vi "DVS_LabVIEWController_one_panel.vi"() -> ()   [LabVIEW 2013]
doc: "This example demonstrates temperature control and monitoring.\n\nNote:\nBefore start this VI is it necessary:\n\n- preconfigure some specific parameters that are not supported by this driver (e.g. PV-I/O Type, Linearization type, Alarm Input Values... ) by Quick Codes, or by Eurotherm iTools or by instrument front panel controls\n- enter correct VISA Resource Descriptor, Device Address and Baud Rate into front-panel controls"
uses:
  <vilib>/Utility/file.llb/Write To Spreadsheet File (string).vi
  <vilib>/Instr/_visa.llb/VISA Configure Serial Port (Instr).vi
  <instrlib>/Keithley 24XX/Public/Data/Read (Single Point).vi
  <instrlib>/Keithley 24XX/Keithley 24XX.lvlib
panel:
  out "Data\nfile\npath":path
  in  "4-wire?":bool
  in  "stop":bool
  in  "Add comments to the   here and click anywhere outside\nthe comment box to save. The time at which the comment is\nsaved is recorded in the data file.":string
  in  "O2 PUMP":bool
  in  "QCM":bool
  in  "Keithley 2420":bool
  in  "J-KEM":bool
  in  "RapidOX":bool
  out "Starting Time":string
  out "Time Elapsed (min)":dbl caption="Elapsed Time (s)"
  in  "Delay Between\nData Points (s)":dbl format="%#_13g"
  in  "Stop after":dbl
  in  "Automatically stop\nmeasurement?":bool
  out "min remaining":dbl
  out "Program Errors":errorcluster
  out "Freq (Hz)":dbl format="%.3e"
  out "R (Ohm)":dbl format="%.3e"
  out "Waveform Chart 7":T1(graph)
  out "Current Temp (C)":dbl
  in  "Setpoint (C)":dbl=25.0
  out "Current Setpoint (C)":dbl
  out "Waveform Chart 5":cluster{dbl, dbl}(graph)
  out "Waveform Chart":cluster{dbl}(graph)
  out "Torr":dbl
  out "%":dbl
  out "atm":dbl
  in  "Com Port":i32(ring) items=["Com 1", "Com 2", "Com 3", "Com 4", "Com 5", "Com 6", "COM 7", "COM 8", "COM 9", "COM 10", "COM 11", "COM 12", "com 13", "COM 14"]
  in  "Baud Rate 2":i32(ring)=2 items=["2400", "4800", "9600", "19200", "38400", "57600", "115200"]
  in  "Com Port 2":i32(ring) items=["Com 1", "Com 2", "Com 3", "Com 4", "Com 5", "Com 6", "COM 7", "COM 8", "COM 9", "COM 10", "COM 11", "COM 12", "com 13", "COM 14"]
  out "Waveform Chart 6":cluster{dbl}(graph)
  out "O2 Concentration (PPM)":dbl
  out "Resistance (Ohm)":sgl
  out "Waveform Chart 4":cluster{"Resistance":sgl}(graph)
  # "Keithley 2420\nRead Resistance"
  # "Setup"
  # "SRS QCM\nController"
  # "Instruments Connected:"
  # "Timing"
  # "Configuring Instrument\n \nPlease Wait......\n\nChart will update in 20 sec"
  # "min"
  # "COMMENT BOX"
  # "J-Kem Temp Control"
  # "Rapidox O2\nSensor"
  # "O2 Partial Pressure"
  # "SetNag\nO2 Pump"
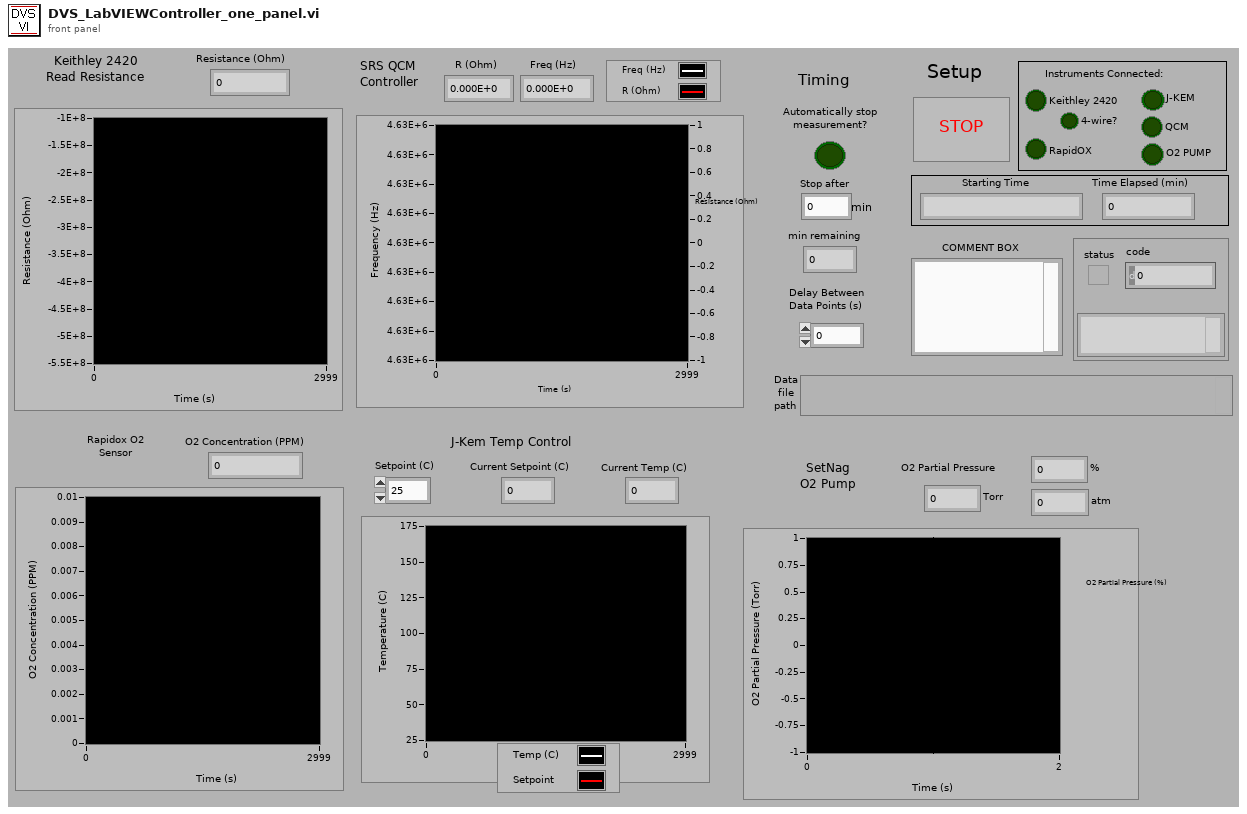
[diagram p1: front panel]
types:
  T1 = cluster{"Frequency out":dbl, "Resistance out":dbl}
  T2 = enum16{"open", "open or create", "create or replace", "create", "open (read only)"}
  T3 = enum16{"no parity", "odd parity", "even parity", "mark parity", "space parity"}
  T4 = cluster{bool, "VISA resource name":refnum<visa-resource-name>, "error out":errorcluster}
  T5 = cluster{bool, "VISA resource name out":refnum<visa-resource-name>, "error out":errorcluster}
  T6 = cluster{"Frequency out":dbl, "Resistance out":dbl}[]
  T7 = cluster{bool, "VISA out":refnum<visa-resource-name>, "error out":errorcluster}
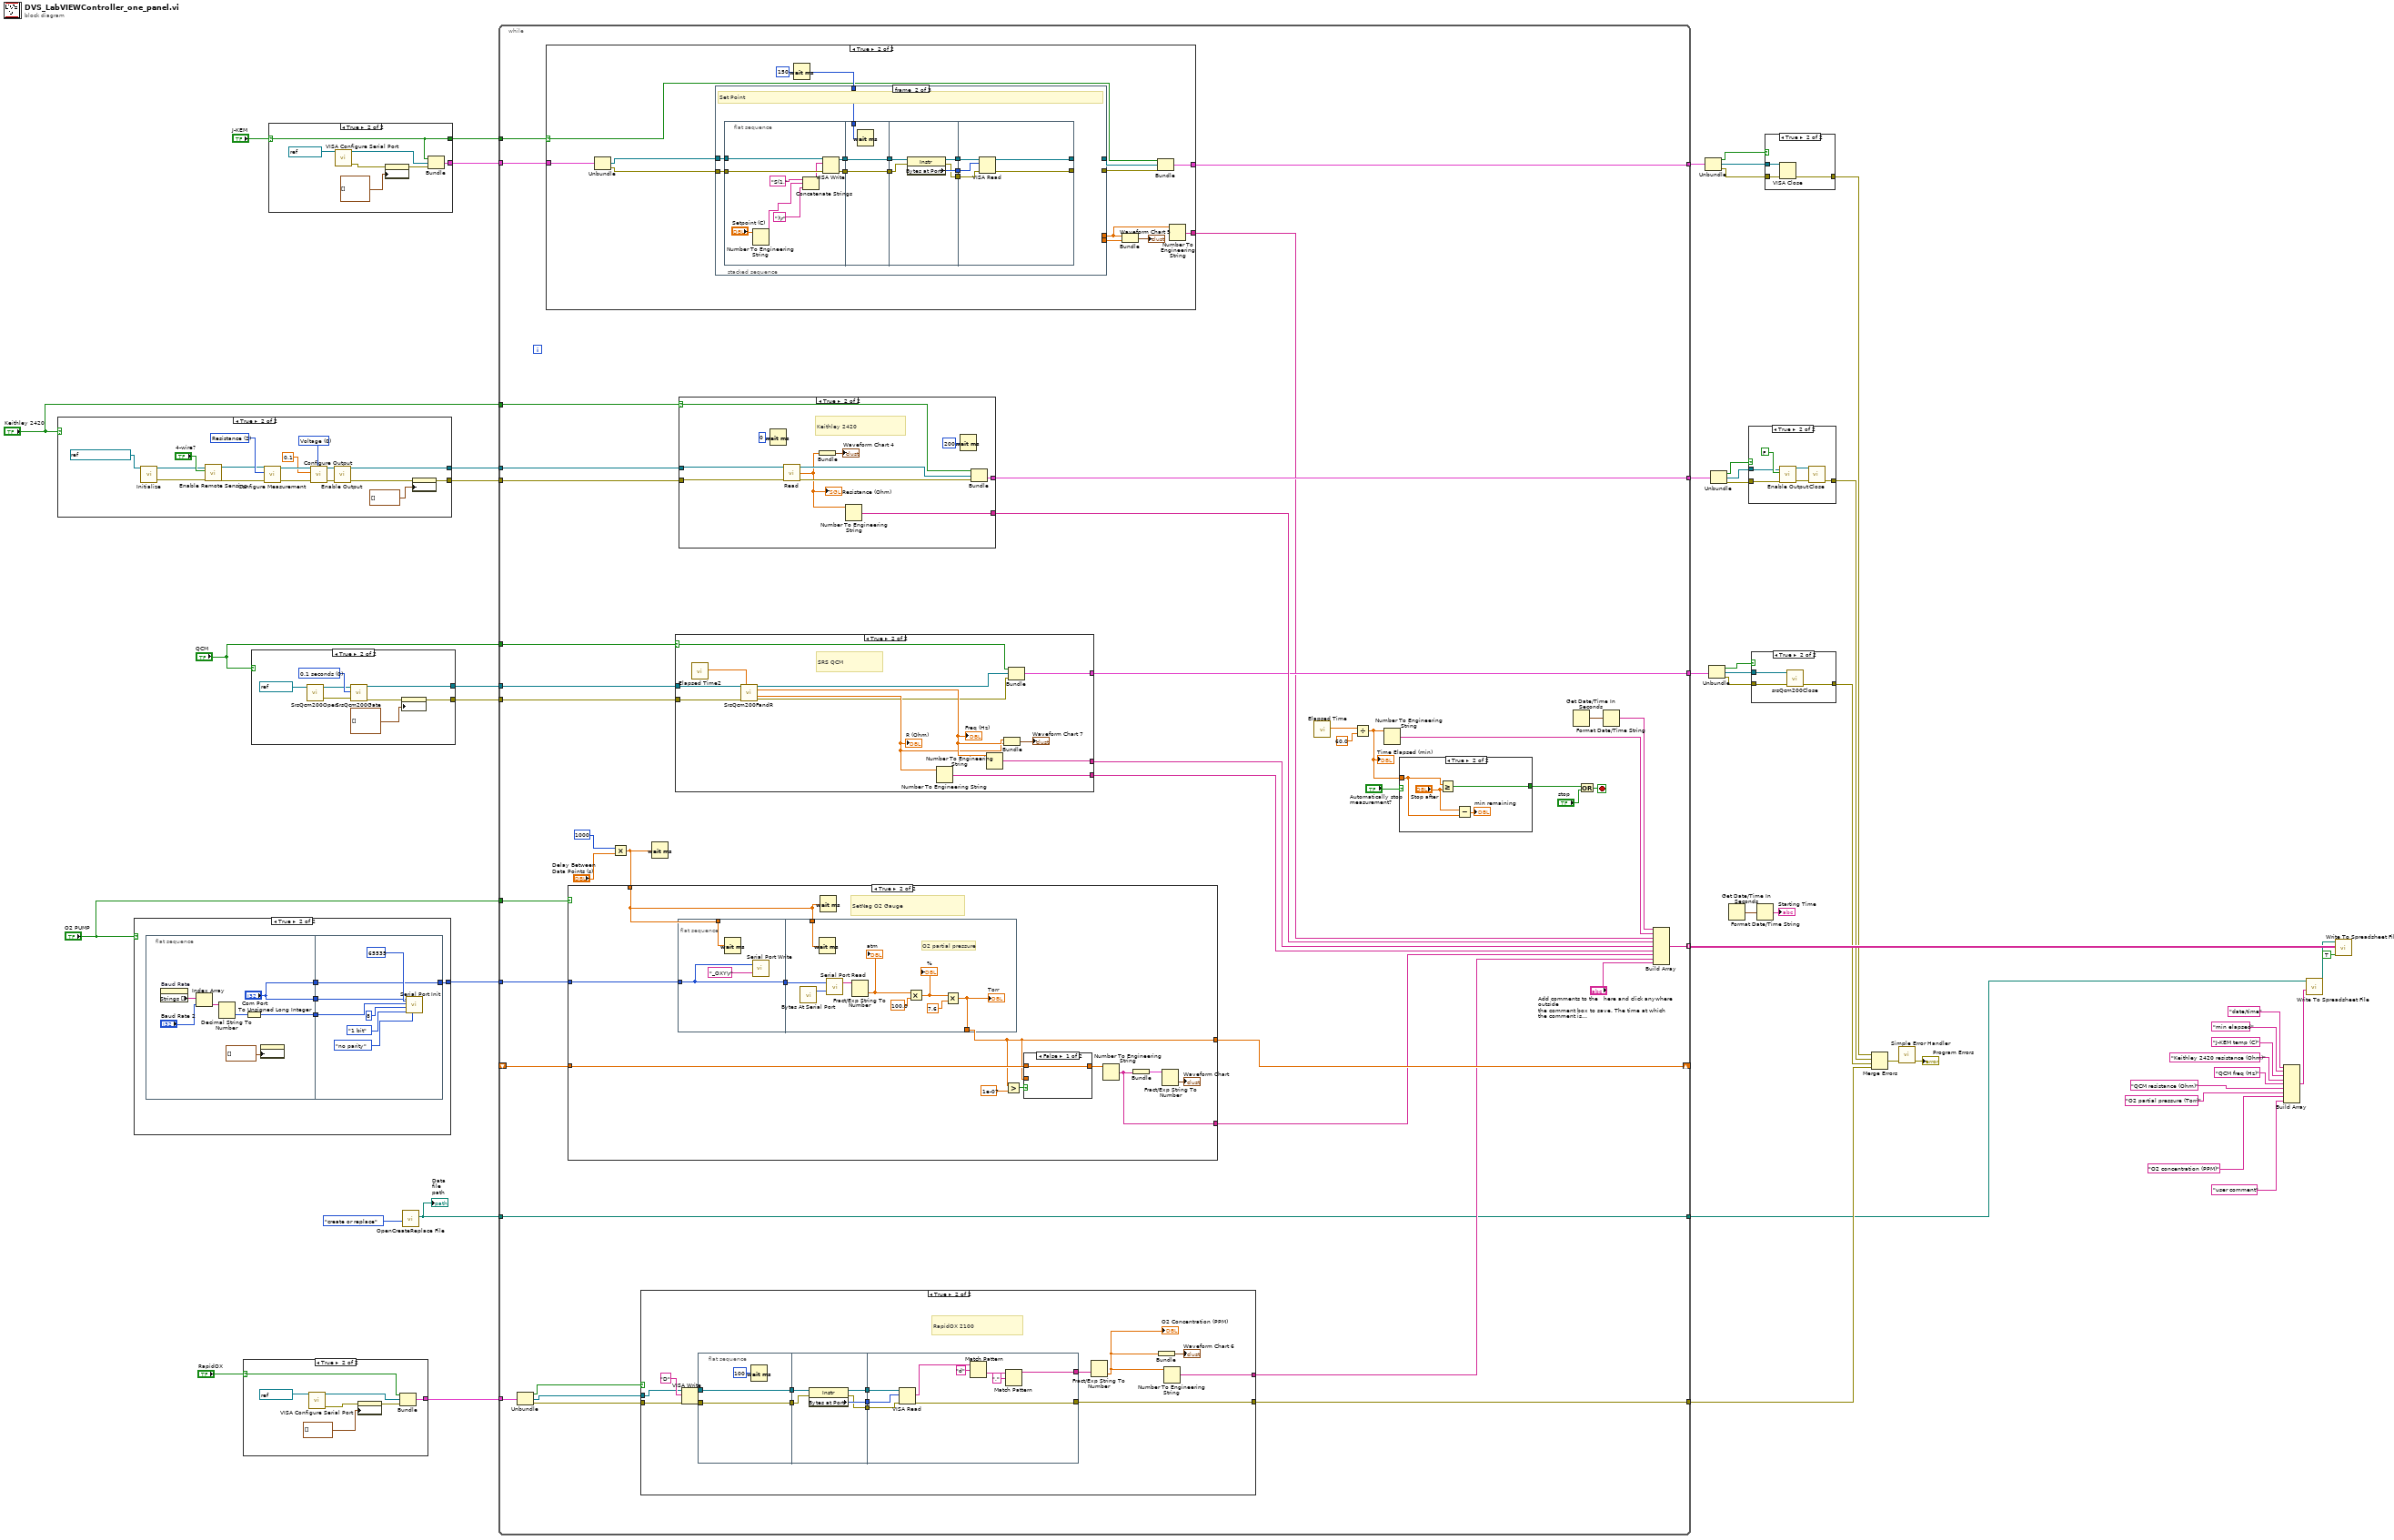
[diagram p0: block diagram]
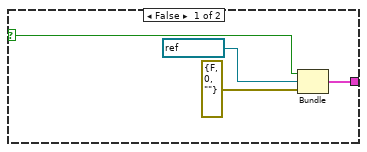
[diagram p2: hidden frame]
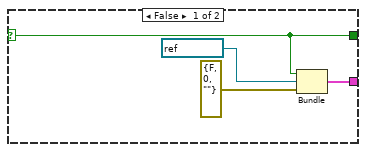
[diagram p4: hidden frame]
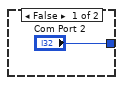
[diagram p5: hidden frame]
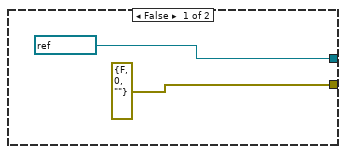
[diagram p7: hidden frame]
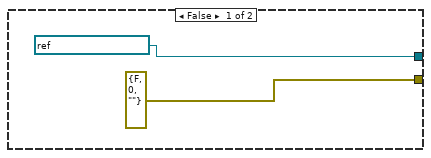
[diagram p9: hidden frame]
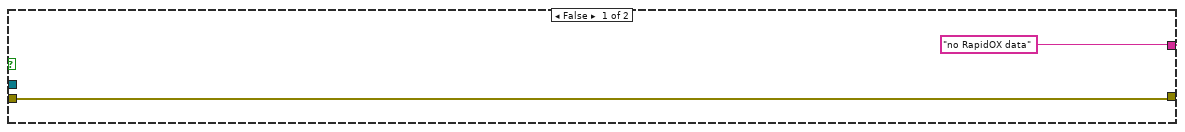
[diagram p10: hidden frame]
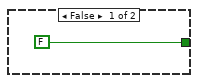
[diagram p11: hidden frame]
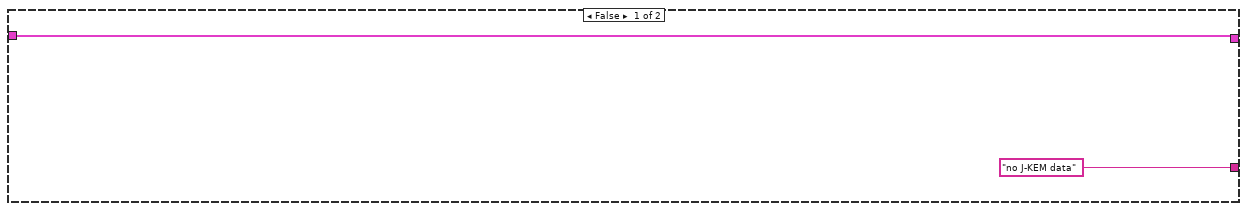
[diagram p12: hidden frame]
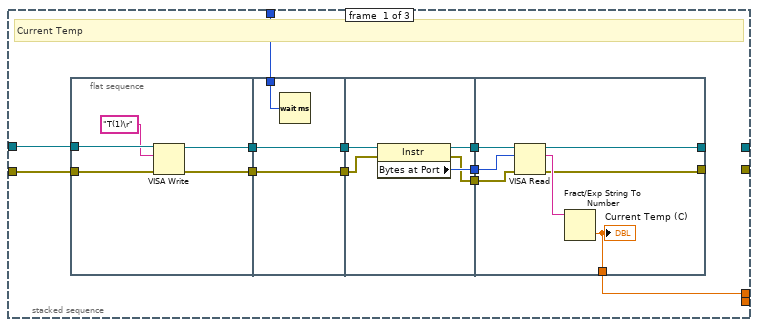
[diagram p13: hidden frame]
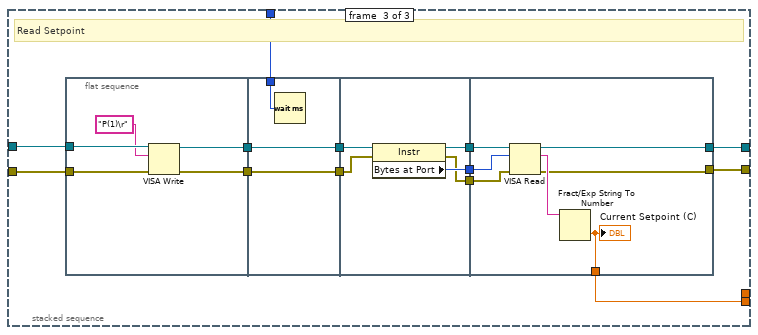
[diagram p14: hidden frame]
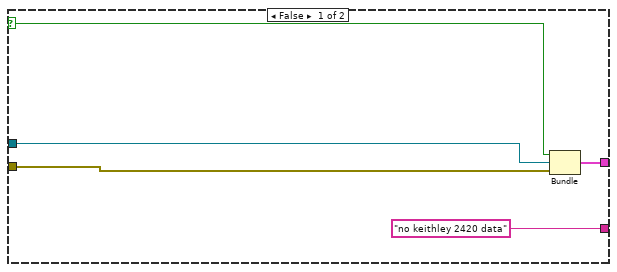
[diagram p15: hidden frame]
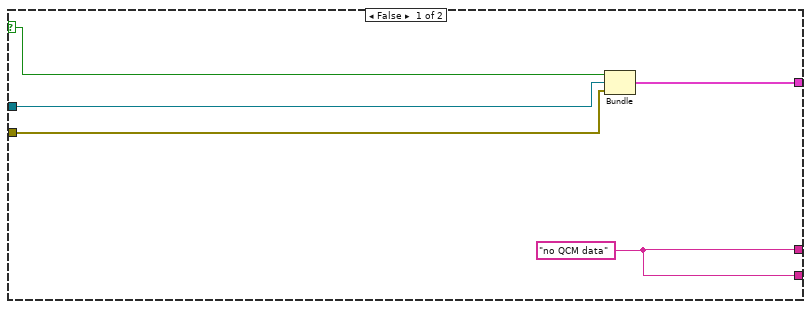
[diagram p16: hidden frame]
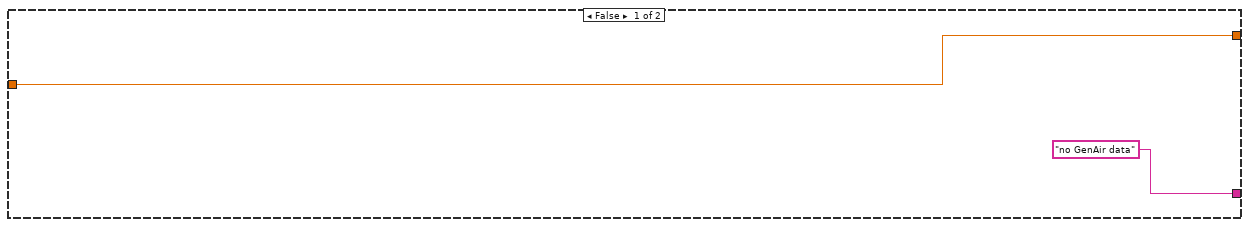
[diagram p17: hidden frame]
diagram:
  n1 = case shown="True" "Keithley 2420" {
    tunnel: [refnum<visa-resource-name> "GPIB1::24::INSTR" ("VISA resource name") w56] -> w43
    tunnel: [errorcluster {"status"=FALSE, "code"=0, "source"=""} ("error out") w59] -> w42
    frame False {
    }
    frame True {
      w62 = u16 0 items=["Voltage", "Current"] ("Source Mode  (0: Voltage)")
      w67 = u16 2 items=["Volts", "Current", "Resistance"] ("Function (0: Volts)")
      n2 = call <instrlib>:"Initialize.vi"("VISA resource name"=refnum<visa-resource-name> "GPIB1::24::INSTR") -> ("error out"=w52:errorcluster, "VISA resource name out"=w55:refnum<visa-resource-name>)  [unwired: 9 in]
      n3 = call <instrlib>:"Enable Remote Sensing.vi"("error in (no error)"=w52, "Enable Remote Sensing (T: Enable)"="4-wire?", "VISA resource name"=w55) -> ("error out"=w53:errorcluster, "VISA resource name out"=w54:refnum<visa-resource-name>)  [unwired: 7 in]
      n4 = call <instrlib>:"Configure Measurement.vi"("error in (no error)"=w53, "Function (0: Volts)"=w67, "VISA resource name"=w54) -> ("error out"=w66:errorcluster, "VISA resource name out"=w65:refnum<visa-resource-name>)  [unwired: 7 in]
      n5 = call <instrlib>:"Configure Output.vi"("Source Mode  (0: Voltage)"=w62, "error in (no error)"=w66, "Output Level (0)"=0.1 ("Output Level (V)"), "VISA resource name"=w65) -> ("error out"=w64:errorcluster, "VISA resource name out"=w63:refnum<visa-resource-name>)  [unwired: 6 in]
      n6 = call <instrlib>:"Enable Output.vi"("error in (no error)"=w64, "VISA resource name"=w63) -> ("error out"=w57:errorcluster, "VISA resource name out"=w56:refnum<visa-resource-name>)  [unwired: 8 in]
      n7 = property on="Waveform Chart 4" class="WFChart (strict)"(error in=w57, "History Data"=cluster{"Resistance":sgl}[] []) -> (error out=w59:errorcluster)  [unwired: 1 in, 1 out]
    }
  }
  n8 = case shown="True" "O2 PUMP" {
    tunnel: ["Com Port 2" w70] -> w37
    frame False {
    }
    frame True {
      n9 = flat-sequence {
        tunnel: ["Com Port"] -> w73
        tunnel: [w76] -> w72
        tunnel: ["Com Port"] -> w71
        tunnel: w73 -> [w82]
        tunnel: w72 -> [w81]
        tunnel: w71 -> [w83]
        tunnel: [w83] -> w70
        frame #0 {
          n10 = property on="Baud Rate" class="Ring (strict)"() -> ("Strings []"=w78:string[])  [unwired: 2 in, 2 out]
          n11 = Index Array(array=w78, index="Baud Rate 2") -> (element=w79:string)
          n12 = Decimal String To Number(string=w79) -> (number=w77:i32)  [unwired: 2 in, 1 out]
          n13 = To Unsigned Long Integer(number=w77) -> (unsigned 32bit integer=w76:u32)
          n14 = property on="Waveform Chart" class="WFChart (strict)"("History Data"=cluster{dbl}[] []) -> ()  [unwired: 2 in, 2 out]
        }
        frame #1 {
          n15 = call <vilib>:"Serial Port Init.vi"("parity"=T3."no parity", "buffer size"=u16 65535, "stop bits"=enum16{"1 bit", "1.5 bits", "2 bits"}."1 bit", "data bits"=u16 8, "baud rate"=w81, "port number"=w82) -> ()  [unwired: 1 in, 1 out]
        }
      }
    }
  }
  n16 = case shown="True" "RapidOX" {
    selector: "RapidOX" -> [w88 w95]
    tunnel: [w89 w96] -> w5
    frame False {
      n17 = Bundle(w88, "VISA resource name"=refnum<visa-resource-name> "COM7", "error out"=errorcluster {"status"=FALSE, "code"=0, "source"=""}) -> (w89:T4)  [unwired: 1 in]
    }
    frame True {
      n18 = call-poly "VISA Configure Serial Port"("VISA resource name"=refnum<visa-resource-name> "COM7") -> ("VISA resource name out"=w97:refnum<visa-resource-name>, "error out"=w93:errorcluster)  [unwired: 13 in]
      n19 = property on="Waveform Chart 6" class="WFChart (strict)"(error in=w93, "History Data"=cluster{dbl}[] []) -> (error out=w92:errorcluster)  [unwired: 1 in, 1 out]
      n20 = Bundle(w95, "VISA resource name out"=w97, "error out"=w92) -> (w96:T5)  [unwired: 1 in]
    }
  }
  n21 = case shown="True" "QCM" {
    tunnel: [refnum<visa-resource-name> "COM6" ("VISA in") w104] -> w41
    tunnel: [errorcluster {"status"=FALSE, "code"=0, "source"=""} ("error out") w102] -> w40
    frame False {
    }
    frame True {
      w108 = u16 0 items=["0.1 seconds", "1.0 seconds", "10.0 seconds"] ("Gate in")
      n22 = call <instrlib>:"SrsQcm200Open.vi"("VISA in"=refnum<visa-resource-name> "COM6") -> ("error out"=w105:errorcluster, "VISA out"=w106:refnum<visa-resource-name>)  [unwired: 4 in]
      n23 = call <instrlib>:"SrsQcm200Gate.vi"("VISA in"=w106, "Gate in"=w108, "error in (no error)"=w105) -> ("VISA out"=w104:refnum<visa-resource-name>, "error out"=w101:errorcluster)  [unwired: 14 in, 1 out]
      n24 = property on="Waveform Chart 7" class="WFChart (strict)"(error in=w101, "History Data"=T6 []) -> (error out=w102:errorcluster)  [unwired: 1 in, 1 out]
    }
  }
  n25 = case shown="True" "J-KEM" {
    selector: "J-KEM" -> [w109 w116]
    tunnel: [w110 w117] -> w26
    tunnel: [w109 w116] -> w19
    frame False {
      n26 = Bundle(w109, "VISA resource name"=refnum<visa-resource-name> "COM3", "error out"=errorcluster {"status"=FALSE, "code"=0, "source"=""}) -> (w110:T4)  [unwired: 1 in]
    }
    frame True {
      n27 = call-poly "VISA Configure Serial Port"("VISA resource name"=refnum<visa-resource-name> "COM3") -> ("VISA resource name out"=w118:refnum<visa-resource-name>, "error out"=w114:errorcluster)  [unwired: 13 in]
      n28 = property on="Waveform Chart 5" class="WFChart (strict)"(error in=w114, "History Data"=cluster{dbl, dbl}[] []) -> (error out=w113:errorcluster)  [unwired: 1 in, 1 out]
      n29 = Bundle(w116, "VISA resource name out"=w118, "error out"=w113) -> (w117:T5)  [unwired: 1 in]
    }
  }
  n30 = call <instrlib>:"OpenCreateReplace File.vi"("function (open:0)"=T2."create or replace") -> ("new file path"=w1:path)  [unwired: 7 in, 3 out]
  "Data\nfile\npath" <- w1
  n31 = while {
    shift-right: [w159] -> _
    shift-left: _ -> [w158]
    tunnel: [w156] -> w45 mode=indexing
    tunnel: "Keithley 2420" -> [w122]
    tunnel: w43 -> [w154]
    tunnel: w42 -> [w153]
    tunnel: w41 -> [w152]
    tunnel: w40 -> [w151]
    tunnel: "QCM" -> [w149]
    tunnel: "O2 PUMP" -> [w142]
    tunnel: w37 -> [w148]
    tunnel: [w144] -> w34
    tunnel: [w143] -> w30
    tunnel: w26 -> [w141]
    tunnel: [w140] -> w24
    tunnel: w19 -> [w138]
    tunnel: w5 -> [w131]
    tunnel: [w126] -> w3
    tunnel: [w120] -> w2
    tunnel: w1 -> [w120]
    stop <- w136 stop-if-true
    n32 = Unbundle(w131) -> (w130:bool, "VISA resource name out"=w129:refnum<visa-resource-name>, "error out"=w128:errorcluster)
    n33 = case shown="True" w138 {
      selector: w138 -> [_ w204]
      tunnel: w141 -> [w202 w209]
      tunnel: [w202 w207] -> w140
      tunnel: ["no J-KEM data" w205] -> w139
      frame False {
      }
      frame True {
        w214 = u32 150 ("milliseconds to wait")
        n34 = Unbundle(w209) -> ("VISA resource name out"=w208:refnum<visa-resource-name>, "error out"=w203:errorcluster)  [unwired: 1 out]
        n35 = stacked-sequence {
          tunnel: w208 -> [w218 w248 w282]
          tunnel: w203 -> [w217 w247 w281]
          tunnel: w214 -> [w216 w246 w283]
          tunnel: [_ _ w280] -> w210
          tunnel: [_ _ w279] -> w211
          tunnel: [w215 _ _] -> w206
          tunnel: [_ _ w278] -> w213
          frame #0 {
            # "Current Temp"
            n36 = flat-sequence {
              tunnel: w218 -> [w230]
              tunnel: w217 -> [w229]
              tunnel: [w227] -> w225
              tunnel: [w226] -> w224
              tunnel: w216 -> [w233]
              tunnel: [w232] -> w223
              tunnel: w225 -> [w232]
              tunnel: w224 -> [w231]
              tunnel: [w231] -> w222
              tunnel: w223 -> [w238]
              tunnel: w222 -> [w237]
              tunnel: [w236] -> w221
              tunnel: [w235] -> w220
              tunnel: [w234] -> w219
              tunnel: w221 -> [w245]
              tunnel: w220 -> [w244]
              tunnel: w219 -> [w243]
              tunnel: [w240] -> _
              tunnel: [w241] -> _
              tunnel: [w239] -> w215
              frame #0 {
                n37 = VISA Write(VISA resource name=w230, write buffer="T(1)\r", error in (no error)=w229) -> (VISA resource name out=w227:refnum<visa-resource-name>, error out=w226:errorcluster)  [unwired: 1 out]
              }
              frame #1 {
                n38 = Wait (ms)(milliseconds to wait=w233) -> ()  [unwired: 1 out]
              }
              frame #2 {
                n39 = property class="Instr"(reference=w238, error in=w237) -> (reference out=w236:refnum<visa-resource-name>, error out=w234:errorcluster, "Bytes at Port"=w235:u32)
              }
              frame #3 {
                n40 = VISA Read(VISA resource name=w245, byte count=w244, error in (no error)=w243) -> (VISA resource name out=w241:refnum<visa-resource-name>, read buffer=w242:string, error out=w240:errorcluster)  [unwired: 1 out]
                n41 = Fract/Exp String To Number(string=w242) -> (number=w239:dbl)  [unwired: 3 in, 1 out]
                "Current Temp (C)" <- w239
              }
            }
          }
          frame #1 {
            # "Set Point"
            n42 = flat-sequence {
              tunnel: w248 -> [w264]
              tunnel: w247 -> [w263]
              tunnel: [w262] -> w255
              tunnel: [w261] -> w254
              tunnel: w246 -> [w267]
              tunnel: [w266] -> w253
              tunnel: w255 -> [w266]
              tunnel: w254 -> [w265]
              tunnel: [w265] -> w252
              tunnel: w253 -> [w272]
              tunnel: w252 -> [w271]
              tunnel: [w270] -> w251
              tunnel: [w269] -> w250
              tunnel: [w268] -> w249
              tunnel: w251 -> [w277]
              tunnel: w250 -> [w276]
              tunnel: w249 -> [w275]
              tunnel: [w273] -> _
              tunnel: [w274] -> _
              frame #0 {
                n43 = Number To Engineering String(4:"Setpoint (C)") -> (0:w257:string)  [unwired: 3 in]
                n44 = Concatenate Strings("S(1," ("write buffer"), w257, ")\r" ("write buffer")) -> (w260:string)
                n45 = VISA Write(VISA resource name=w264, write buffer=w260, error in (no error)=w263) -> (VISA resource name out=w262:refnum<visa-resource-name>, error out=w261:errorcluster)  [unwired: 1 out]
              }
              frame #1 {
                n46 = Wait (ms)(milliseconds to wait=w267) -> ()  [unwired: 1 out]
              }
              frame #2 {
                n47 = property class="Instr"(reference=w272, error in=w271) -> (reference out=w270:refnum<visa-resource-name>, error out=w268:errorcluster, "Bytes at Port"=w269:u32)
              }
              frame #3 {
                n48 = VISA Read(VISA resource name=w277, byte count=w276, error in (no error)=w275) -> (VISA resource name out=w274:refnum<visa-resource-name>, error out=w273:errorcluster)  [unwired: 2 out]
              }
            }
          }
          frame #2 {
            # "Read Setpoint"
            n49 = flat-sequence {
              tunnel: w282 -> [w295]
              tunnel: w281 -> [w294]
              tunnel: [w292] -> w290
              tunnel: [w291] -> w289
              tunnel: [w298] -> w288
              tunnel: w290 -> [w298]
              tunnel: w289 -> [w297]
              tunnel: [w297] -> w287
              tunnel: w283 -> [w296]
              tunnel: w288 -> [w303]
              tunnel: w287 -> [w302]
              tunnel: [w301] -> w286
              tunnel: [w300] -> w285
              tunnel: [w299] -> w284
              tunnel: w286 -> [w310]
              tunnel: w285 -> [w309]
              tunnel: w284 -> [w308]
              tunnel: [w305] -> w279
              tunnel: [w306] -> w280
              tunnel: [w304] -> w278
              frame #0 {
                n50 = VISA Write(VISA resource name=w295, write buffer="P(1)\r", error in (no error)=w294) -> (VISA resource name out=w292:refnum<visa-resource-name>, error out=w291:errorcluster)  [unwired: 1 out]
              }
              frame #1 {
                n51 = Wait (ms)(milliseconds to wait=w296) -> ()  [unwired: 1 out]
              }
              frame #2 {
                n52 = property class="Instr"(reference=w303, error in=w302) -> (reference out=w301:refnum<visa-resource-name>, error out=w299:errorcluster, "Bytes at Port"=w300:u32)
              }
              frame #3 {
                n53 = VISA Read(VISA resource name=w310, byte count=w309, error in (no error)=w308) -> (VISA resource name out=w306:refnum<visa-resource-name>, read buffer=w307:string, error out=w305:errorcluster)  [unwired: 1 out]
                n54 = Fract/Exp String To Number(string=w307) -> (number=w304:dbl)  [unwired: 3 in, 1 out]
                "Current Setpoint (C)" <- w304
              }
            }
          }
        }
        n55 = Wait (ms)(milliseconds to wait=w214) -> ()  [unwired: 1 out]
        n56 = Bundle(w206, w213) -> (→"Waveform Chart 5":cluster{dbl, dbl})  [unwired: 1 in]
        n57 = Bundle(w204, "VISA resource name out"=w210, "error out"=w211) -> (w207:T5)  [unwired: 1 in]
        n58 = Number To Engineering String(4:w206) -> (0:w205:string)  [unwired: 3 in]
      }
    }
    n59 = Multiply(x=u32 1000, y="Delay Between\nData Points (s)") -> (x*y=w125:dbl)
    n60 = case shown="True" w142 {
      tunnel: [w345 w349] -> w159
      tunnel: w158 -> [w345 w350]
      tunnel: w125 -> [_ w346]
      tunnel: w148 -> [_ w348]
      tunnel: ["no GenAir data" w347] -> w147
      frame False {
      }
      frame True {
        # "SetNag O2 Gauge"
        n61 = flat-sequence {
          tunnel: [w359] -> w356
          tunnel: w346 -> [w361]
          tunnel: w348 -> [w359]
          tunnel: w356 -> [w362]
          tunnel: w346 -> [w369]
          tunnel: [w365] -> w349
          frame #0 {
            n62 = Wait (ms)(milliseconds to wait=w361) -> ()  [unwired: 1 out]
            n63 = call <vilib>:"Serial Port Write.vi"("string to write"="_OXY\r" ("O2 partial press"), "port number"=w359) -> ()  [unwired: 1 out]
          }
          frame #1 {
            # "O2 partial pressure"
            n64 = call <vilib>:"Bytes At Serial Port.vi"() -> ("byte count"=w370:u32)  [unwired: 1 in, 1 out]
            n65 = Wait (ms)(milliseconds to wait=w369) -> ()  [unwired: 1 out]
            n66 = call <vilib>:"Serial Port Read.vi"("requested byte count"=w370, "port number"=w362) -> ("string read"=w368:string)  [unwired: 1 out]
            n67 = Fract/Exp String To Number(string=w368) -> (number=w366:dbl)  [unwired: 3 in, 1 out]
            "atm" <- w366
            n68 = Multiply(x=w366, y=100.0) -> (x*y=w363:dbl)
            "%" <- w363
            n69 = Multiply(x=w363, y=7.6) -> (x*y=w365:dbl)
            "Torr" <- w365
          }
        }
        n70 = Wait (ms)(milliseconds to wait=w346) -> ()  [unwired: 1 out]
        n71 = Greater?(x=w349, y=1e-07) -> (0:w352:bool)
        n72 = case shown="False" w352 {
          tunnel: [w357 w358] -> w351
          tunnel: w349 -> [_ w358]
          tunnel: w350 -> [w357 _]
          frame False {
          }
          frame True {
          }
        }
        n73 = Number To Engineering String(4:w351) -> (0:w347:string)  [unwired: 3 in]
        n74 = Bundle(w347) -> (w354:cluster{string})  [unwired: 1 in]
        n75 = Fract/Exp String To Number(string=w354) -> (number=→"Waveform Chart":cluster{dbl})  [unwired: 3 in, 1 out]
      }
    }
    n76 = case shown="True" w130 {
      tunnel: w129 -> [_ w169]
      tunnel: w128 -> [w162 w168]
      tunnel: ["no RapidOX data" w167] -> w127
      tunnel: [w162 w164] -> w126
      frame False {
      }
      frame True {
        # "RapidOX 2100"
        n77 = VISA Write(VISA resource name=w169, write buffer="D", error in (no error)=w168) -> (VISA resource name out=w172:refnum<visa-resource-name>, error out=w171:errorcluster)  [unwired: 1 out]
        n78 = flat-sequence {
          tunnel: [w181] -> w178
          tunnel: [w179] -> w177
          tunnel: w172 -> [w181]
          tunnel: w171 -> [w179]
          tunnel: w178 -> [w186]
          tunnel: w177 -> [w185]
          tunnel: [w184] -> w176
          tunnel: [w183] -> w175
          tunnel: [w182] -> w174
          tunnel: w176 -> [w195]
          tunnel: w175 -> [w194]
          tunnel: w174 -> [w193]
          tunnel: [w192] -> w164
          tunnel: [w187] -> w166
          frame #0 {
            n79 = Wait (ms)(milliseconds to wait=u32 100) -> ()  [unwired: 1 out]
          }
          frame #1 {
            n80 = property class="Instr"(reference=w186, error in=w185) -> (reference out=w184:refnum<visa-resource-name>, error out=w182:errorcluster, "Bytes at Port"=w183:u32)
          }
          frame #2 {
            n81 = VISA Read(VISA resource name=w195, byte count=w194, error in (no error)=w193) -> (read buffer=w190:string, error out=w192:errorcluster)  [unwired: 2 out]
            n82 = Match Pattern(string=w190, regular expression="d") -> (after substring=w188:string)  [unwired: 1 in, 3 out]
            n83 = Match Pattern(string=w188, regular expression=",") -> (before substring=w187:string)  [unwired: 1 in, 3 out]
          }
        }
        n84 = Fract/Exp String To Number(string=w166) -> (number=w165:dbl)  [unwired: 3 in, 1 out]
        "O2 Concentration (PPM)" <- w165
        n85 = Bundle(w165) -> (→"Waveform Chart 6":cluster{dbl})  [unwired: 1 in]
        n86 = Number To Engineering String(4:w165) -> (0:w167:string)  [unwired: 3 in]
      }
    }
    n87 = Wait (ms)(milliseconds to wait=w125) -> ()  [unwired: 1 out]
    n88 = case shown="True" w149 {
      selector: w149 -> [w330 w337]
      tunnel: w152 -> [w329 w342]
      tunnel: w151 -> [w328 w341]
      tunnel: [w331 w340] -> w150
      tunnel: [w331 w339] -> w146
      tunnel: [w327 w336] -> w143
      frame False {
        w331 = "no QCM data"
        n89 = Bundle(w330, "VISA out"=w329, "error out"=w328) -> (w327:T7)  [unwired: 1 in]
      }
      frame True {
        # "SRS QCM"
        n90 = call "Elapsed Time2"() -> ("Elapsed Time (s)"=w343:dbl)  [unwired: 12 in, 7 out]
        n91 = call <instrlib>:"SrsQcm200FandR.vi"("VISA in"=w342, "Reference time in"=w343, "error in (no error)"=w341) -> ("VISA out"=w338:refnum<visa-resource-name>, "Frequency out"=w334:dbl, "Resistance out"=w333:dbl, "error out"=w332:errorcluster)  [unwired: 6 in, 3 out]
        "Freq (Hz)" <- w334
        "R (Ohm)" <- w333
        n92 = Number To Engineering String(4:w333) -> (0:w339:string)  [unwired: 3 in]
        n93 = Number To Engineering String(4:w334) -> (0:w340:string)  [unwired: 3 in]
        n94 = Bundle("Frequency out"=w334, "Resistance out"=w333) -> (→"Waveform Chart 7":T1)  [unwired: 1 in]
        n95 = Bundle(w337, "VISA out"=w338, "error out"=w332) -> (w336:T7)  [unwired: 1 in]
      }
    }
    n96 = case shown="True" w122 {
      selector: w122 -> [w314 w323]
      tunnel: w154 -> [w313 w317]
      tunnel: w153 -> [w312 w316]
      tunnel: [w311 w321] -> w144
      tunnel: ["no keithley 2420 data" w320] -> w145
      frame False {
        n97 = Bundle(w314, "VISA resource name out"=w313, "error out"=w312) -> (w311:T5)  [unwired: 1 in]
      }
      frame True {
        # "Keithley 2420"
        n98 = Wait (ms)(milliseconds to wait=u32 0) -> ()  [unwired: 1 out]
        n99 = call-poly <instrlib>:"Read.vi"("VISA resource name"=w317, "error in (no error)"=w316) -> ("VISA resource name out"=w324:refnum<visa-resource-name>, "Resistance"=w318:sgl, "error out"=w322:errorcluster)  [unwired: 7 in, 4 out]
        "Resistance (Ohm)" <- w318
        n100 = Bundle("Resistance"=w318) -> (→"Waveform Chart 4":cluster{"Resistance":sgl})  [unwired: 1 in]
        n101 = Number To Engineering String(4:w318) -> (0:w320:string)  [unwired: 3 in]
        n102 = Wait (ms)(milliseconds to wait=u32 200) -> ()  [unwired: 1 out]
        n103 = Bundle(w323, "VISA resource name out"=w324, "error out"=w322) -> (w321:T5)  [unwired: 1 in]
      }
    }
    n104 = call "Elapsed Time"() -> ("Elapsed Time (s)"=w135:dbl)  [unwired: 12 in, 7 out]
    n105 = Divide(x=w135, y=60.0) -> (x/y=w121:dbl)
    "Time Elapsed (min)" <- w121
    n106 = Number To Engineering String(4:w121) -> (0:w160:string)  [unwired: 3 in]
    n107 = case shown="True" "Automatically stop\nmeasurement?" {
      tunnel: w121 -> [_ w198]
      tunnel: [FALSE w200] -> w132
      frame False {
      }
      frame True {
        n108 = Greater Or Equal?(x=w198, y="Stop after") -> (x >= y?=w200:bool)
        n109 = Subtract(x="Stop after", y=w198) -> (x-y=→"min remaining":dbl)
      }
    }
    n110 = Get Date/Time In Seconds() -> (seconds since 1Jan1904=w161:timestamp)
    n111 = Or(x=w132, y="stop") -> (x .or. y?=w136:bool)
    n112 = Format Date/Time String(seconds (now)=w161) -> (date/time string=w155:string)  [unwired: 2 in]
    n113 = Build Array(w155, w160, w139, w145, w150, w146, w147, w127, "Add comments to the   here and click anywhere outside\nthe comment box to save. The time at which the comment is\nsaved is recorded in the data file.") -> (w156:string[])
  }
  n114 = Unbundle(w24) -> (w23:bool, "VISA resource name out"=w22:refnum<visa-resource-name>, "error out"=w21:errorcluster)
  n115 = Unbundle(w30) -> (w29:bool, "VISA out"=w28:refnum<visa-resource-name>, "error out"=w27:errorcluster)
  n116 = Unbundle(w34) -> (w33:bool, "VISA resource name out"=w32:refnum<visa-resource-name>, "error out"=w31:errorcluster)
  n117 = Get Date/Time In Seconds() -> (seconds since 1Jan1904=w48:timestamp)
  n118 = case shown="True" w33 {
    tunnel: w32 -> [_ w374]
    tunnel: w31 -> [w371 w373]
    tunnel: [w371 w372] -> w35
    frame False {
    }
    frame True {
      n119 = call <instrlib>:"Enable Output.vi"("error in (no error)"=w373, "Enable Output (T: Enable)"=FALSE, "VISA resource name"=w374) -> ("error out"=w375:errorcluster, "VISA resource name out"=w377:refnum<visa-resource-name>)  [unwired: 7 in]
      n120 = call <instrlib>:"Close.vi"("error in (no error)"=w375, "VISA resource name"=w377) -> ("error out"=w372:errorcluster)  [unwired: 9 in]
    }
  }
  n121 = case shown="True" w29 {
    tunnel: w27 -> [w378 w381]
    tunnel: [w378 w380] -> w36
    tunnel: w28 -> [_ w379]
    frame False {
    }
    frame True {
      n122 = call <instrlib>:"srsQcm200Close.vi"("error in"=w381, "Visa in"=w379) -> ("error out"=w380:errorcluster)  [unwired: 3 in]
    }
  }
  n123 = Format Date/Time String(seconds (now)=w48) -> (date/time string=→"Starting Time":string)  [unwired: 2 in]
  n124 = case shown="True" w23 {
    tunnel: w22 -> [_ w385]
    tunnel: w21 -> [w382 w384]
    tunnel: [w382 w383] -> w20
    frame False {
    }
    frame True {
      n125 = VISA Close(VISA resource name=w385, error in (no error)=w384) -> (error out=w383:errorcluster)
    }
  }
  n126 = Merge Errors(w20, w35, w36, w3) -> (w46:errorcluster)
  n127 = call <vilib>:"Simple Error Handler.vi"("error in (no error)"=w46) -> ("error out"=→"Program Errors":errorcluster)  [unwired: 4 in, 4 out]
  n128 = Build Array("date/time", "min elapsed", "J-KEM temp (C)", "Keithley 2420 resistance (Ohm)" ("element"), "QCM freq (Hz)", "QCM resistance (Ohm)", "O2 partial pressure (Torr)" ("element"), "O2 concentration (PPM)" ("element"), "user comment" ("element")) -> (w11:string[])
  n129 = call-poly <vilib>:"Write To Spreadsheet File.vi"("1D data"=w11, "file path (dialog if empty)"=w2) -> ("new file path (Not A Path if cancelled)"=w12:path)  [unwired: 6 in]
  n130 = call-poly <vilib>:"Write To Spreadsheet File.vi"("append to file? (new file:F)"=TRUE, "2D data"=w45, "file path (dialog if empty)"=w12) -> ()  [unwired: 5 in, 1 out]
